vi "SQL Execute.vi"(8 "error in (no error)":errorcluster, 10 "Command Text":string, 11 "DataBase_SQL in":refnum<class "DataBase_SQL.lvclass">) -> (0 "error out":errorcluster, 1 "FirstRow":string[](array[string]), 2 "Datas":string[][](table), 3 "DataBase_SQL out":refnum<class "DataBase_SQL.lvclass">, 4 "Rows Fetched":i32)   [LabVIEW 2021, in "DataBase_SQL.lvclass"]
uses:
  <userlib>/John_Lib/DataBase/DataBase_SQL/DataBase_SQL.lvclass
  <userlib>/John_Lib/DataBase/DataBase_SQL/DataBase_SQL.lvclass/DataBase_SQL.ctl
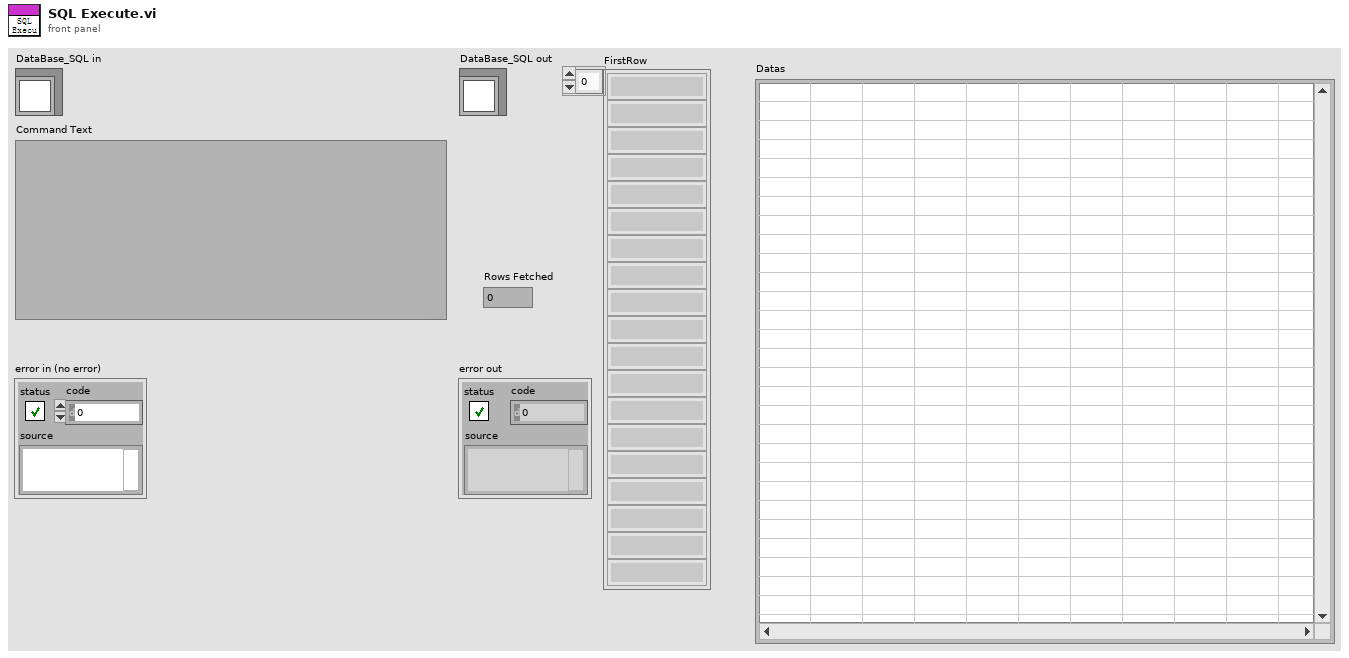
[diagram p1: front panel]
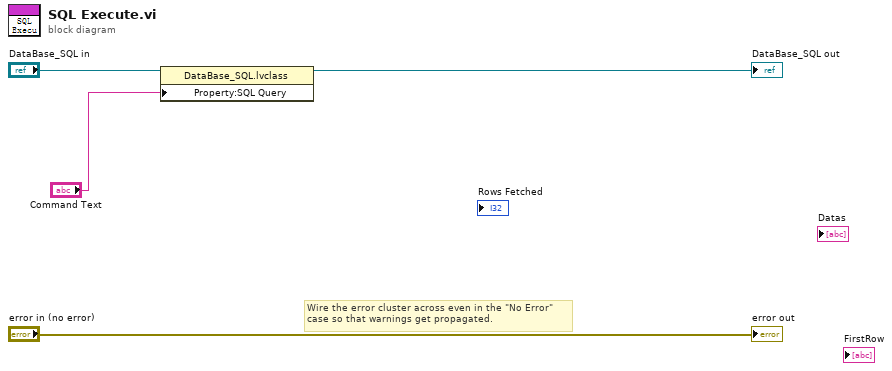
[diagram p0: block diagram]
diagram:
  # "Wire the error cluster across even in the \"No Error\"\ncase so that warnings get propagated."
  n1 = property class="DataBase_SQL.lvclass"(reference="DataBase_SQL in", "Property:SQL Query"="Command Text") -> (reference out=→"DataBase_SQL out":refnum<class "DataBase_SQL.lvclass">)  [unwired: 1 in, 1 out]
  "error out" <- "error in (no error)"
